vi "FGV_Current_Evens.vi"(0 "new events":T1[](array[typedef])) -> (4 "CurrentEvents":T1[](array[typedef]))   [LabVIEW 2019, in "Logger.lvclass"]
uses:
  Logger.lvclass
  EventData.ctl
  TypeDef/AlarmType.ctl
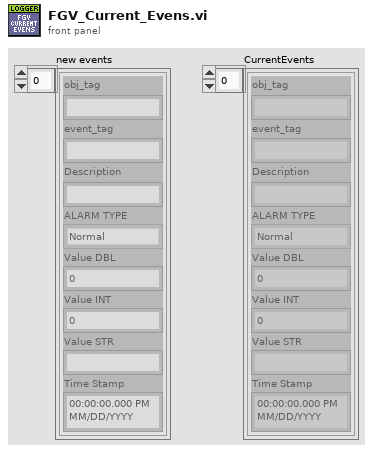
[diagram p1: front panel]
types:
  T1 = typedef "EventData.ctl" = cluster{"obj_tag":string, "event_tag":string, "Description":string, "ALARM TYPE":T2, "Value DBL":dbl, "Value INT":i32, "Value STR":string, "Time Stamp":timestamp}
  T2 = typedef "AlarmType.ctl" = enum16{"Normal", "Warning", "Alarm"}
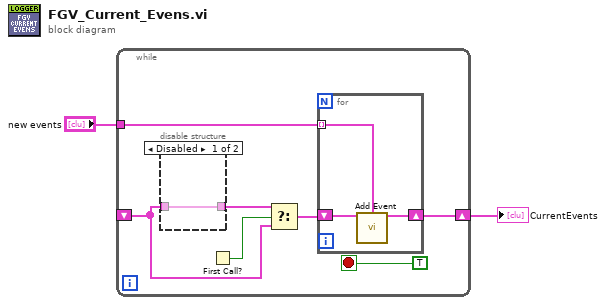
[diagram p0: block diagram]
diagram:
  n1 = while {
    tunnel: "new events" -> [w9]
    shift-right: [w8] -> w1
    shift-left: _ -> [w6]
    stop <- TRUE stop-if-true
    n2 = disable-structure shown="Disabled" {
      disable-tunnel: w6 -> [w10 _]
      disable-tunnel: [w10 _] -> w5
      frame Disabled {
      }
      frame Enabled {
      }
    }
    n3 = First Call?() -> (First Call?: T/F=w7:bool)
    n4 = Select(t=w5, s=w7, f=w6) -> (s? t:f=w4:T1[])
    n5 = for {
      tunnel: w9 -> [w11] mode=indexing
      shift-right: [w13] -> w8
      shift-left: w4 -> [w12]
      n6 = call "Add Event.vi"("CurrentEvents In"=w12, "Event"=w11) -> ("CurrentEvents out"=w13:T1[])  [unwired: 13 in]
    }
  }
  "CurrentEvents" <- w1
